vi "reload_settings.vi"(8 "error in (no error)":errorcluster, 11 "TrajectoryMH100122AODRAPS in":refnum<class "TrajectoryMH100122AODRAPS.lvclass">) -> (0 "error out":errorcluster, 3 "TrajectoryMH100122AODRAPS out":refnum<class "TrajectoryMH100122AODRAPS.lvclass">)   [LabVIEW 2010, in "TrajectoryMH100122AODRAPS.lvclass"]
uses:
  TrajectoryMH100122AODRAPS.lvclass
  common/xcontrols/XImage/XImage/XImage.xctl
  class_data.vi
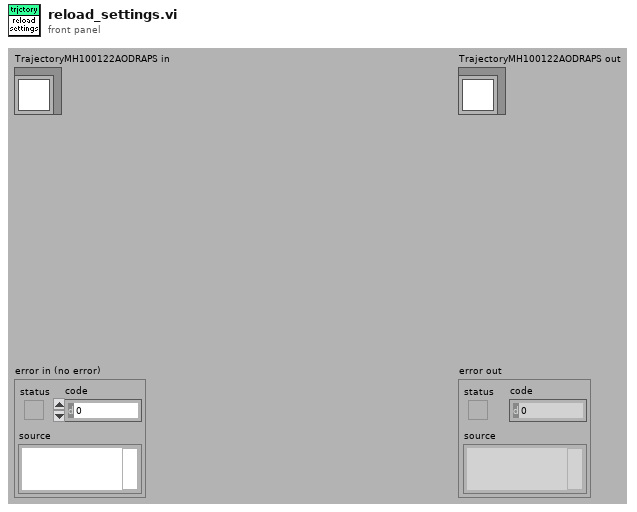
[diagram p1: front panel]
types:
  T1 = typedef "TrajectoryMH100122AODRAPS.lvclass/settings_cluster.ctl" = cluster{"no. of points":i32, "pixel dwell time":dbl[unit], "transformation factors":dbl[unit][], "2p imaging mirror switch":bool, "no. of frames":i32, "x resolution":u32, "zoom":dbl, "z angle (rotation angle, phi)":dbl[unit], "x angle (tilting angle, phi)":dbl[unit], "offset":dbl[unit][], "sub-pattern?":bool, "spiral radius":i8, "motion correction array size":u8, "y resolution":u32, "extrapolate line size":i32, "ROI color":u32, "line points color":u32, "z-step size / frame":u16, "z-offset":u16, "ROI numbering":bool, "winding number":dbl, "number of iteration points":dbl, "height":dbl, "amp":dbl}
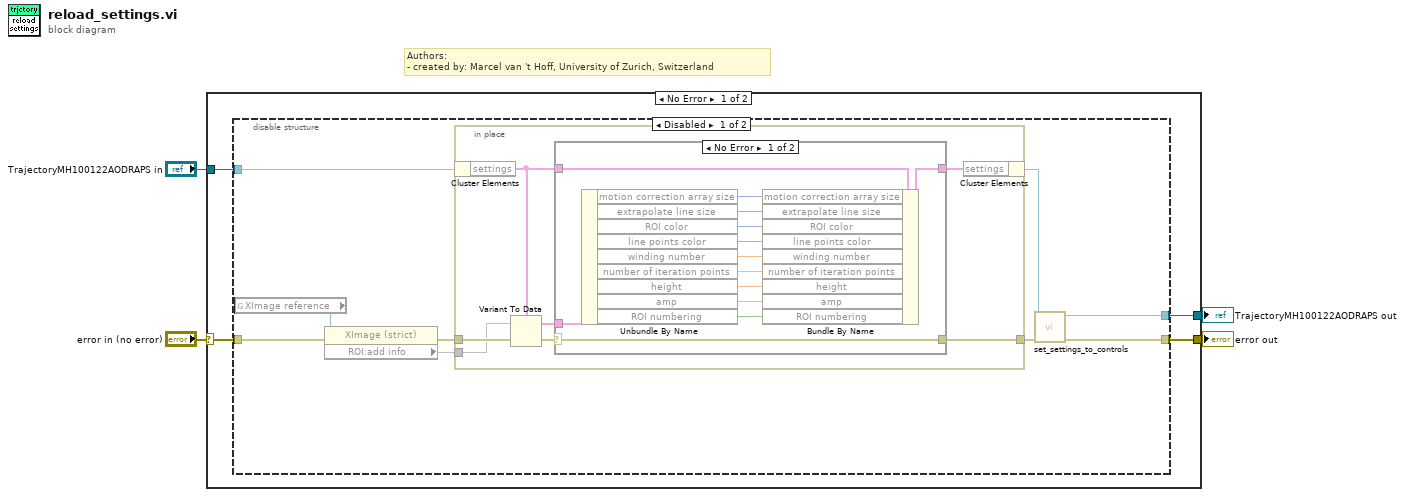
[diagram p0: block diagram]
diagram:
  # "Authors: \n- created by: Marcel van 't Hoff, University of Zurich, Switzerland"
  n1 = case shown="No Error" "error in (no error)" {
    selector: "error in (no error)" -> [w6 w42]
    tunnel: [w5 w42] -> w3
    tunnel: [w7 w41] -> w1
    tunnel: "TrajectoryMH100122AODRAPS in" -> [w8 w41]
    frame No Error {
      n2 = disable-structure shown="Disabled" {
        disable-tunnel: w8 -> [w14 w40]
        disable-tunnel: [w13 w40] -> w7
        disable-tunnel: w6 -> [w11 w39]
        disable-tunnel: [w10 w39] -> w5
        frame Disabled {
          n3 = global read "class_data.vi" "XImage reference"() -> (w9:refnum<vi>)
          n4 = property class="XImage (strict)"(reference=w9, error in=w11) -> (error out=w16:errorcluster, "ROI:add info"=w17)  [unwired: 1 out]
          n5 = in-place {
            in-place-border: [w18] -> w12
            in-place-border: w16 -> [w24]
            in-place-border: w17 -> [w23]
            n6 = in-place-cluster #1(w14) -> ("settings"=w22:T1)
            n7 = Variant To Data(error in=w24, Variant=w23, type=w22) -> (error out=w19:errorcluster, data=w20:T1)
            n8 = case shown="No Error" w19 {
              selector: w19 -> [w27 _]
              tunnel: w22 -> [w37 w38]
              tunnel: [w36 w38] -> w21
              tunnel: w20 -> [w35 _]
              tunnel: [w27 _] -> w18
              frame No Error {
                n9 = Unbundle By Name(w35) -> ("motion correction array size"=w34:u8, "extrapolate line size"=w33:i32, "ROI color"=w32:u32, "line points color"=w31:u32, "winding number"=w30:dbl, "number of iteration points"=w29:dbl, "height"=w26:dbl, "amp"=w25:dbl, "ROI numbering"=w28:bool)
                n10 = Bundle By Name(cluster=w37, "motion correction array size"=w34, "extrapolate line size"=w33, "ROI color"=w32, "line points color"=w31, "winding number"=w30, "number of iteration points"=w29, "height"=w26, "amp"=w25, "ROI numbering"=w28) -> (w36:T1)
              }
              frame Error {
              }
            }
            n11 = in-place-cluster #1("settings"=w21) -> (w15:refnum<class "TrajectoryMH100122AODRAPS.lvclass">)
          }
          n12 = call-dynamic "set_settings_to_controls.vi"("error in (no error)"=w12, "TrajectoryMH100122AODRAPS in"=w15) -> ("error out"=w10:errorcluster, "TrajectoryMH100122AODRAPS out"=w13:refnum<class "TrajectoryMH100122AODRAPS.lvclass">)  [unwired: 8 in]
        }
        frame Enabled {
        }
      }
    }
    frame Error {
    }
  }
  "error out" <- w3
  "TrajectoryMH100122AODRAPS out" <- w1
